vi "Test Cases - API String Arguments Support(Variant).vi"() -> ()   [LabVIEW 2017]
uses:
  API-String-Arugments-Support/API String Arguments Support.lvlib
panel:
  in  "String 12":string="[3.12,4.113,2.3,5;3.12,5,2.3;3.12,4.11,5]"
  out "error 12":errorcluster
  out "Data 11":dbl[][](array[numeric])=[[3.12, 4.113, 2.3, 5.0, 5.0, 2.3, 4.11, 5.0]]
  in  "String 11":string="[{Bool:Off;child.name:ddd},{Bool:On;name:ddd}]"
  out "error 11":errorcluster
  out "Data 10":T1(array[cluster])=[{"Name"="", "Child"={"Name"="ddd"}, "Bool"=FALSE}, {"Name"="ddd", "Child"={"Name"=""}, "Bool"=TRUE}]
  in  "String 10":string="C:\\ni-rt\\data\\a\\2023.07.25"
  out "error 10":errorcluster
  out "Data 9":path=path "C:/ni-rt/data/a/2023.07.25"
  in  "String 9":string="Bool:Off;child.name:ddd"
  out "error 9":errorcluster
  out "Data 8":T2={"Name"="abc", "Child"={"Name"="ddd"}, "Bool"=FALSE}
  in  "String 8":string="[3.12,4.11,5]"
  out "error 8":errorcluster
  out "Data 4":dbl[](array[numeric])=[3.12, 4.11, 5.0]
  in  "String 7":string="ccccc"
  out "error 7":errorcluster
  out "Data 7":enum16{"1 - aaaa", "2 - bbbb", "555 - ccccc"}(ring)=enum."555 - ccccc"
  in  "String 6":string="555"
  out "error 6":errorcluster
  out "Data 6":enum16{"1 - aaaa", "2 - bbbb", "555 - ccccc"}(ring)=enum."555 - ccccc"
  in  "String 5":string="bbbb"
  out "error 5":errorcluster
  out "Data 5":enum16{"aaaa", "bbbb", "ccccc"}(ring)=enum."bbbb"
  in  "String 4":string="3.1415926"
  out "error 4":errorcluster
  out "Data 4":dbl=3.1415926
  in  "String 3":string="0x42"
  out "error 3":errorcluster
  out "Data 3":i32=66
  in  "String 2":string="Enable"
  out "error 2":errorcluster
  out "Data 2":bool=TRUE
  out "Data 1":string="abcd"
  out "error 1":errorcluster
  in  "String":string="abcd"
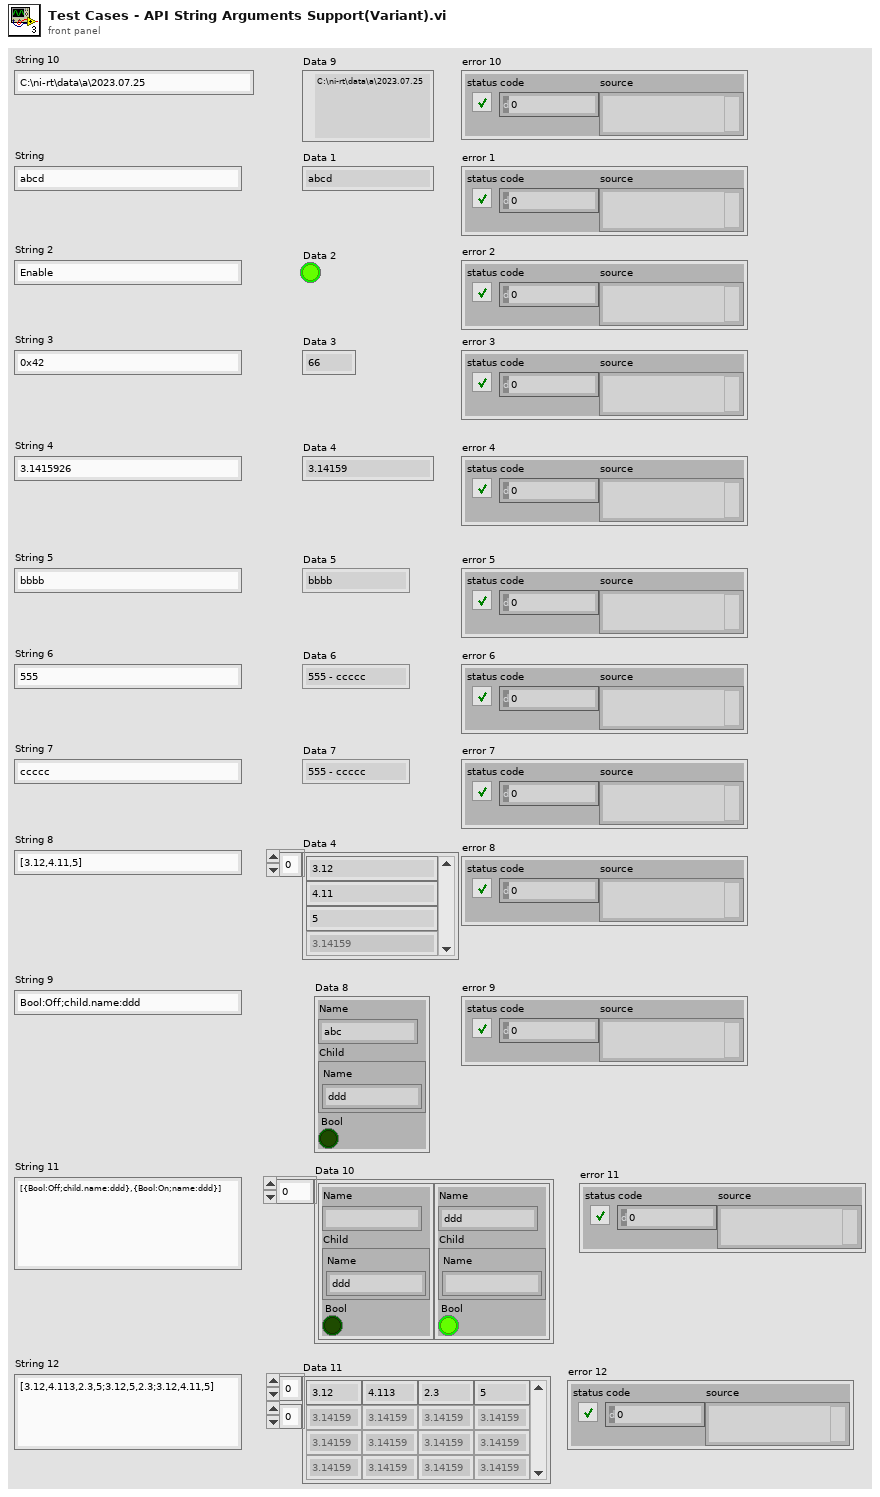
[diagram p1: front panel]
types:
  T1 = cluster{"Name":string, "Child":cluster{"Name":string}, "Bool":bool}[]
  T2 = cluster{"Name":string, "Child":cluster{"Name":string}, "Bool":bool}
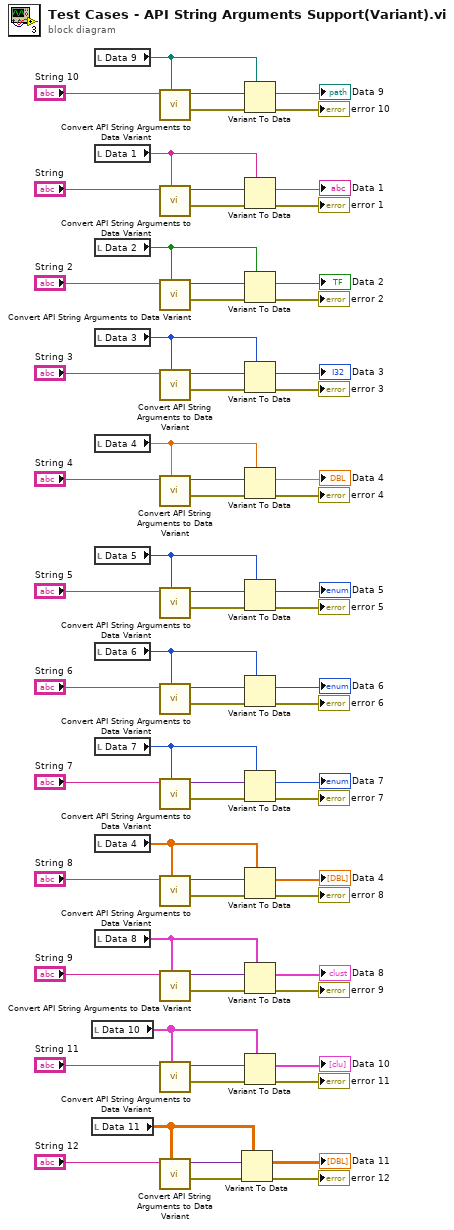
[diagram p0: block diagram]
diagram:
  n1 = local read "Data 10"() -> (w9:T1)
  n2 = local read "Data 11"() -> (w1:dbl[][])
  n3 = local read "Data 9"() -> (w15:path)
  n4 = local read "Data 1"() -> (w70:string)
  n5 = local read "Data 2"() -> (w69:bool)
  n6 = local read "Data 3"() -> (w64:i32)
  n7 = local read "Data 4"() -> (w63:dbl)
  n8 = local read "Data 5"() -> (w58:enum16{"aaaa", "bbbb", "ccccc"})
  n9 = local read "Data 6"() -> (w57:enum16{"1 - aaaa", "2 - bbbb", "555 - ccccc"})
  n10 = local read "Data 7"() -> (w52:enum16{"1 - aaaa", "2 - bbbb", "555 - ccccc"})
  n11 = local read "Data 4"() -> (w51:dbl[])
  n12 = local read "Data 8"() -> (w46:T2)
  n13 = call "Convert API String Arguments to Data Variant.vi"("Type"=w15, "String"="String 10") -> ("error"=w17:errorcluster, "Data"=w16:variant)  [unwired: 8 in]
  n14 = call "Convert API String Arguments to Data Variant.vi"("Type"=w70, "String"="String") -> ("error"=w20:errorcluster, "Data"=w21:variant)  [unwired: 8 in]
  n15 = call "Convert API String Arguments to Data Variant.vi"("Type"=w69, "String"="String 2") -> ("error"=w44:errorcluster, "Data"=w43:variant)  [unwired: 8 in]
  n16 = call "Convert API String Arguments to Data Variant.vi"("Type"=w64, "String"="String 3") -> ("error"=w41:errorcluster, "Data"=w42:variant)  [unwired: 8 in]
  n17 = call "Convert API String Arguments to Data Variant.vi"("Type"=w63, "String"="String 4") -> ("error"=w39:errorcluster, "Data"=w40:variant)  [unwired: 8 in]
  n18 = call "Convert API String Arguments to Data Variant.vi"("Type"=w58, "String"="String 5") -> ("error"=w37:errorcluster, "Data"=w38:variant)  [unwired: 8 in]
  n19 = call "Convert API String Arguments to Data Variant.vi"("Type"=w57, "String"="String 6") -> ("error"=w35:errorcluster, "Data"=w36:variant)  [unwired: 8 in]
  n20 = call "Convert API String Arguments to Data Variant.vi"("Type"=w52, "String"="String 7") -> ("error"=w33:errorcluster, "Data"=w34:variant)  [unwired: 8 in]
  n21 = call "Convert API String Arguments to Data Variant.vi"("Type"=w51, "String"="String 8") -> ("error"=w31:errorcluster, "Data"=w32:variant)  [unwired: 8 in]
  n22 = call "Convert API String Arguments to Data Variant.vi"("Type"=w46, "String"="String 9") -> ("error"=w29:errorcluster, "Data"=w30:variant)  [unwired: 8 in]
  n23 = call "Convert API String Arguments to Data Variant.vi"("Type"=w9, "String"="String 11") -> ("error"=w11:errorcluster, "Data"=w10:variant)  [unwired: 8 in]
  n24 = call "Convert API String Arguments to Data Variant.vi"("Type"=w1, "String"="String 12") -> ("error"=w5:errorcluster, "Data"=w4:variant)  [unwired: 8 in]
  n25 = Variant To Data(error in=w5, type=w1, Variant=w4) -> (data=→"Data 11":dbl[][], error out=→"error 12":errorcluster)
  n26 = Variant To Data(error in=w17, type=w15, Variant=w16) -> (data=→"Data 9":path, error out=→"error 10":errorcluster)
  n27 = Variant To Data(error in=w20, type=w70, Variant=w21) -> (data=→"Data 1":string, error out=→"error 1":errorcluster)
  n28 = Variant To Data(error in=w44, type=w69, Variant=w43) -> (data=→"Data 2":bool, error out=→"error 2":errorcluster)
  n29 = Variant To Data(error in=w41, type=w64, Variant=w42) -> (data=→"Data 3":i32, error out=→"error 3":errorcluster)
  n30 = Variant To Data(error in=w39, type=w63, Variant=w40) -> (data=→"Data 4":dbl, error out=→"error 4":errorcluster)
  n31 = Variant To Data(error in=w37, type=w58, Variant=w38) -> (data=→"Data 5":enum16{"aaaa", "bbbb", "ccccc"}, error out=→"error 5":errorcluster)
  n32 = Variant To Data(error in=w35, type=w57, Variant=w36) -> (data=→"Data 6":enum16{"1 - aaaa", "2 - bbbb", "555 - ccccc"}, error out=→"error 6":errorcluster)
  n33 = Variant To Data(error in=w33, type=w52, Variant=w34) -> (data=→"Data 7":enum16{"1 - aaaa", "2 - bbbb", "555 - ccccc"}, error out=→"error 7":errorcluster)
  n34 = Variant To Data(error in=w31, type=w51, Variant=w32) -> (data=→"Data 4":dbl[], error out=→"error 8":errorcluster)
  n35 = Variant To Data(error in=w29, type=w46, Variant=w30) -> (data=→"Data 8":T2, error out=→"error 9":errorcluster)
  n36 = Variant To Data(error in=w11, type=w9, Variant=w10) -> (data=→"Data 10":T1, error out=→"error 11":errorcluster)
